vi "005 Aleatori.vi"() -> ()   [LabVIEW 2019]
uses:
  <vilib>/numeric/Random Number (Range) DBL.vi
panel:
  in  "stop 2":bool
  in  "Boolean":bool
  out "Resultat 2":dbl format="%#_4g"
  out "Número Aleatori 2":dbl
  in  "Divisor 2":dbl
  in  "Genera nombre aleatori\nentre 5 i 25":bool
  in  "stop":bool
  out "Resultat":dbl format="%#_4g"
  out "Número Aleatori":dbl
  in  "Divisor":dbl
  # "EXEMPLE DE CASE EVENT"
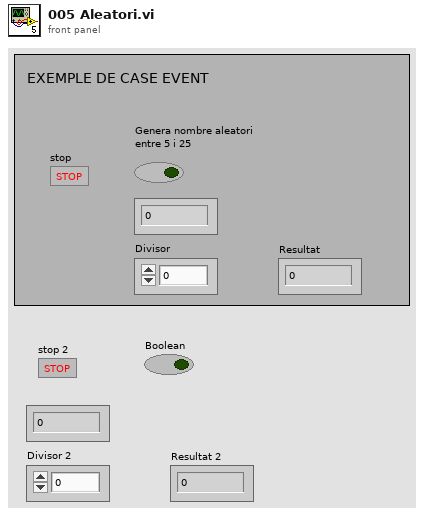
[diagram p1: front panel]
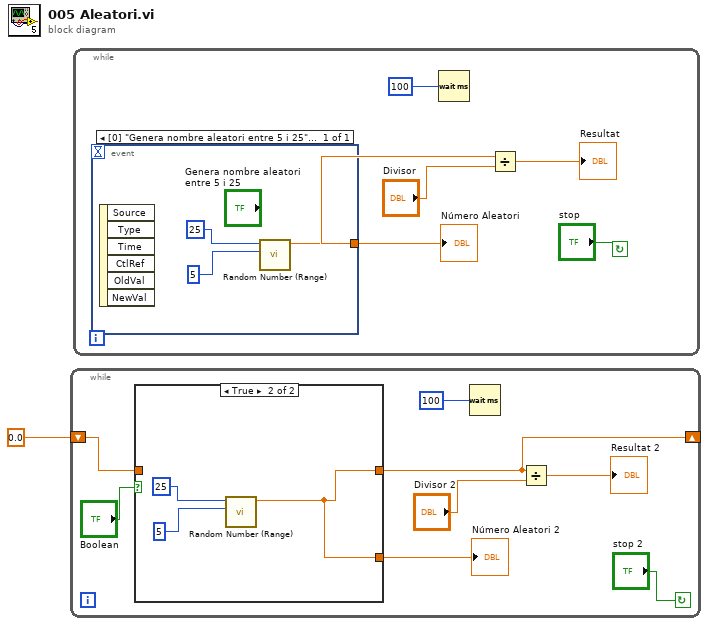
[diagram p0: block diagram]
diagram:
  n1 = while {
    shift-right: [w5] -> _
    shift-left: 0.0 -> [w4]
    stop <- "stop 2" continue-if-true
    n2 = case shown="True" "Boolean" {
      tunnel: [w10 w11] -> w6
      tunnel: [w10 w11] -> w5
      tunnel: w4 -> [w10 _]
      frame False {
      }
      frame True {
        n3 = call-poly <vilib>:"Random Number (Range).vi"("lower bound (0)"=5, "upper bound (100)"=25) -> ("number"=w11:dbl)  [unwired: 9 in]
      }
    }
    "Número Aleatori 2" <- w6
    n4 = Wait (ms)(milliseconds to wait=100) -> ()  [unwired: 1 out]
    n5 = Divide(x=w5, y="Divisor 2") -> (x/y=→"Resultat 2":dbl)
  }
  n6 = while {
    stop <- "stop" continue-if-true
    n7 = event shown="[0] \"Genera nombre aleatori entre 5 i 25\": Value Change" {
      selector: _ -> [_]
      dyn-events: _ -> [_]
      timeout: _ -> [_]
      tunnel: [w19] -> w14
      event "Genera nombre aleatori\nentre 5 i 25": Value Change {
        n8 = event-data() -> ()  [unwired: 1 in, 6 out]
        n9 = call-poly <vilib>:"Random Number (Range).vi"("lower bound (0)"=5, "upper bound (100)"=25) -> ("number"=w19:dbl)  [unwired: 9 in]
      }
    }
    "Número Aleatori" <- w14
    n10 = Wait (ms)(milliseconds to wait=100) -> ()  [unwired: 1 out]
    n11 = Divide(x=w14, y="Divisor") -> (x/y=→"Resultat":dbl)
  }
